vi "oax_Generate Simulated Two Channel Data.vi"(11 "scaled signals [EU]":waveform(dbl)[](array[waveform])) -> (3 "scaled signals [EU] out":waveform(dbl)[](array[waveform]))   [LabVIEW 2017]
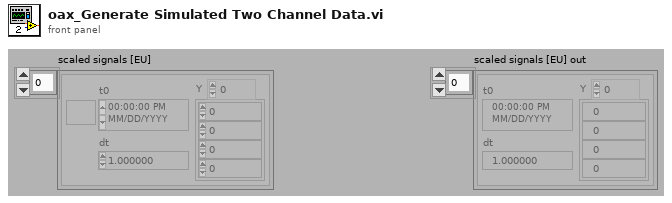
[diagram p1: front panel]
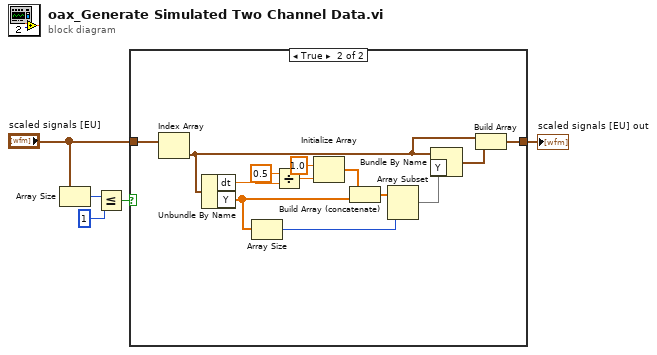
[diagram p0: block diagram]
diagram:
  n1 = Array Size(array="scaled signals [EU]") -> (size(s)=w5:i32)
  n2 = Less Or Equal?(x=w5, y=1) -> (x <= y?=w3:bool)
  n3 = case shown="True" w3 {
    tunnel: "scaled signals [EU]" -> [w6 w19]
    tunnel: [w6 w7] -> w1
    frame False {
    }
    frame True {
      n4 = Index Array(array=w19) -> (element=w8:waveform(dbl))  [unwired: 1 in]
      n5 = Unbundle By Name(w8) -> ("dt"=w18:dbl, "Y"=w13:dbl[])
      n6 = Array Size(array=w13) -> (size(s)=w11:i32)
      n7 = Divide(x=0.5, y=w18) -> (x/y=w16:dbl)
      n8 = Initialize Array(1.0 ("element"), w16) -> (w14:dbl[])
      n9 = Build Array (concatenate)(w14, w13) -> (w12:dbl[])
      n10 = Array Subset(array=w12, length=w11) -> (w10:dbl[])  [unwired: 1 in]
      n11 = Bundle By Name(cluster=w8, "Y"=w10) -> (w9:waveform(dbl))
      n12 = Build Array(w8, w9) -> (w7:waveform(dbl)[])
    }
  }
  "scaled signals [EU] out" <- w1
